vi "Table Constructor Adv Schema DB.vi"(8 "error in (no error)":errorcluster, 9 "Table Name":string, 10 "Database":refnum<class "Database Adv Schema.lvclass">, 11 "Table Configuration Adv Schema DB in":refnum<class "Table Configuration Adv Schema DB.lvclass">) -> (0 "error out":errorcluster, 3 "Table Configuration Adv Schema DB out":refnum<class "Table Configuration Adv Schema DB.lvclass">)   [LabVIEW 2020, in "Table.lvlib" / "Table Configuration Adv Schema DB.lvclass"]
uses:
  Table Configuration Adv Schema DB.lvclass
  C:/Users/User/Desktop/Raman Program/Database OOP/source/Database OOP/Table Configuration/Table Configuration.lvclass
  Database Interfaces/Database Advanced Schema Class/Database Adv Schema.lvclass
  Table Configuration Adv Schema DB.lvclass/Table Configuration Adv Schema DB.ctl
  Table Configuration/Table Configuration.lvclass/Table Configuration.ctl
  Table Configuration/Table Configuration.lvclass
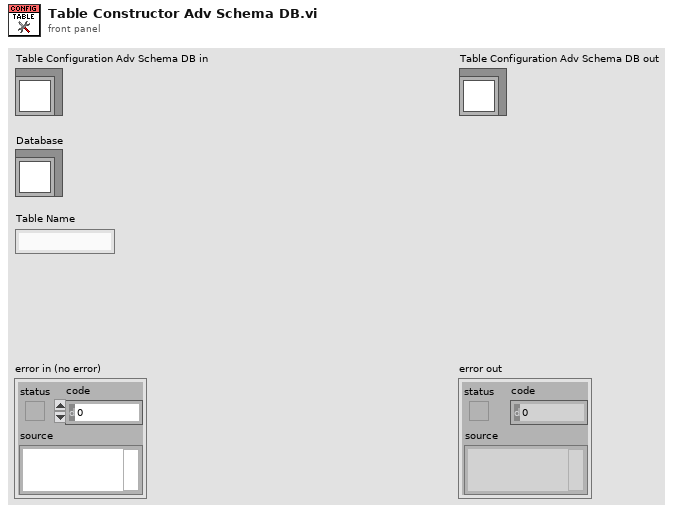
[diagram p1: front panel]
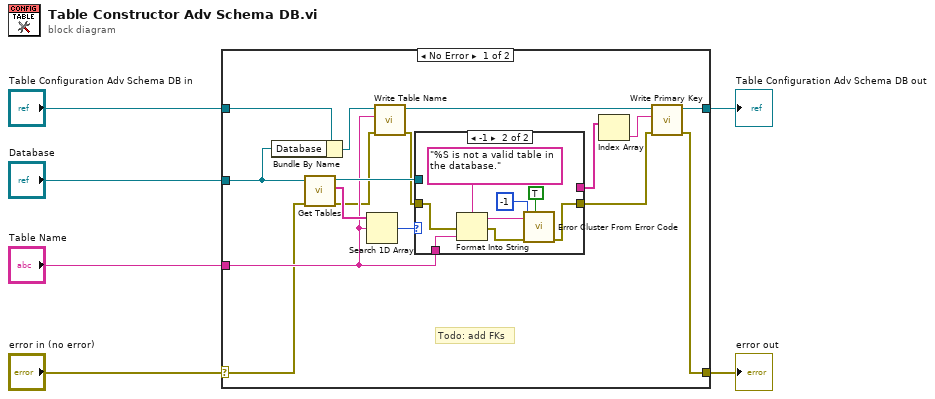
[diagram p0: block diagram]
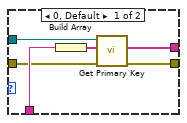
[diagram p2: hidden frame]
diagram:
  n1 = case shown="No Error" "error in (no error)" {
    selector: "error in (no error)" -> [w11 w38]
    tunnel: [w10 w38] -> w5
    tunnel: [w9 w37] -> w3
    tunnel: "Table Configuration Adv Schema DB in" -> [w18 w37]
    tunnel: "Database" -> [w22 _]
    tunnel: "Table Name" -> [w15 _]
    frame No Error {
      # "Todo: add FKs"
      n2 = Bundle By Name(cluster=w18, "Database"=w22) -> (w8:refnum<class "Table Configuration Adv Schema DB.lvclass">)
      n3 = call-dynamic "Get Tables.vi"("error in (no error)"=w11, "Database Interface in"=w22) -> ("error out"=w14:errorcluster, "Table Names"=w21:string[], "Database Interface out"=w19:refnum<class "Database Adv Schema.lvclass">)  [unwired: 7 in]
      n4 = Search 1D Array(1D array=w21, element=w15) -> (index of element=w20:i32)  [unwired: 1 in]
      n5 = call "Write Table Name.vi"("error in (no error)"=w14, "Table Name"=w15, "Table Configuration in"=w8) -> ("error out"=w13:errorcluster, "Table Configuration out"=w7:refnum<class "Table Configuration Adv Schema DB.lvclass">)  [unwired: 7 in]
      n6 = case shown="-1" w20 {
        tunnel: w19 -> [w28 _]
        tunnel: w15 -> [w27 w36]
        tunnel: w13 -> [w25 w31]
        tunnel: [w24 w29] -> w12
        tunnel: [w23 _] -> w17
        frame 0, Default {
          n7 = Build Array(w27) -> (w26:string[])
          n8 = call-dynamic "Get Primary Key.vi"("error in (no error)"=w25, "Table Name Array"=w26, "Database Schema in"=w28) -> ("error out"=w24:errorcluster, "Primary Key Array"=w23:string[])  [unwired: 5 in, 2 out]
        }
        frame -1 {
          n9 = Format Into String(format string="%S is not a valid table in the database.", error in=w31, w36) -> (resulting string=w34:string, error out=w30:errorcluster)  [unwired: 1 in]
          n10 = call <vilib>:"Error Cluster From Error Code.vi"("show call chain? (False)"=TRUE, "error in (no error)"=w30, "error message (\"\")"=w34, "error code (0)"=-1) -> ("error out"=w29:errorcluster)  [unwired: 5 in]
        }
      }
      n11 = Index Array(array=w17) -> (element=w16:string)  [unwired: 1 in]
      n12 = call "Write Primary Key.vi"("error in (no error)"=w12, "Primary Key"=w16, "Table Configuration in"=w7) -> ("error out"=w10:errorcluster, "Table Configuration out"=w9:refnum<class "Table Configuration Adv Schema DB.lvclass">)  [unwired: 7 in]
    }
    frame Error {
    }
  }
  "error out" <- w5
  "Table Configuration Adv Schema DB out" <- w3
